vi "update two devices.vi"(0 "VISA resource name":refnum<visa-resource-name>, 7 "Firmware file for Master":path, 11 "Firmware file for Screen":path) -> (15 "error out":errorcluster)   [LabVIEW 2010]
uses:
  <vilib>/Instr/_visa.llb/VISA Configure Serial Port (Instr).vi
panel:
  out "Slide 2":dbl(slide) scale=0.0..1.0
  out "Pages to program 2":T1(array[cluster])
  out "Slide":dbl(slide) scale=0.0..1.0
  out "Pages to program":T1(array[cluster])
  # "Master's Firmware"
  # "Screen's Firmware"
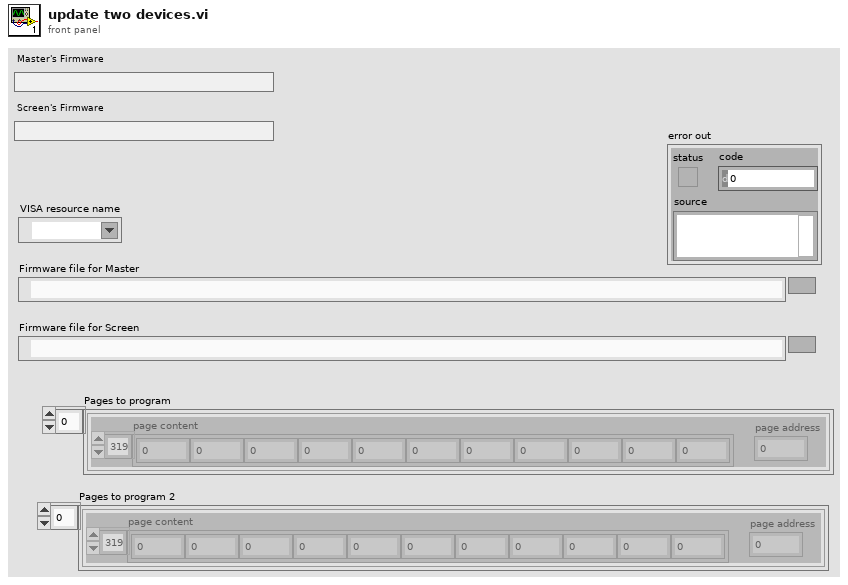
[diagram p1: front panel]
types:
  T1 = cluster{"page content":u8[], "page address":u32}[]
  T2 = cluster{"Byte count":u8, "Address":u16, "Record Type":u8, "Data":u8[], "Checksum":u8, "Start code":string, "Checksum (my)":u8}[]
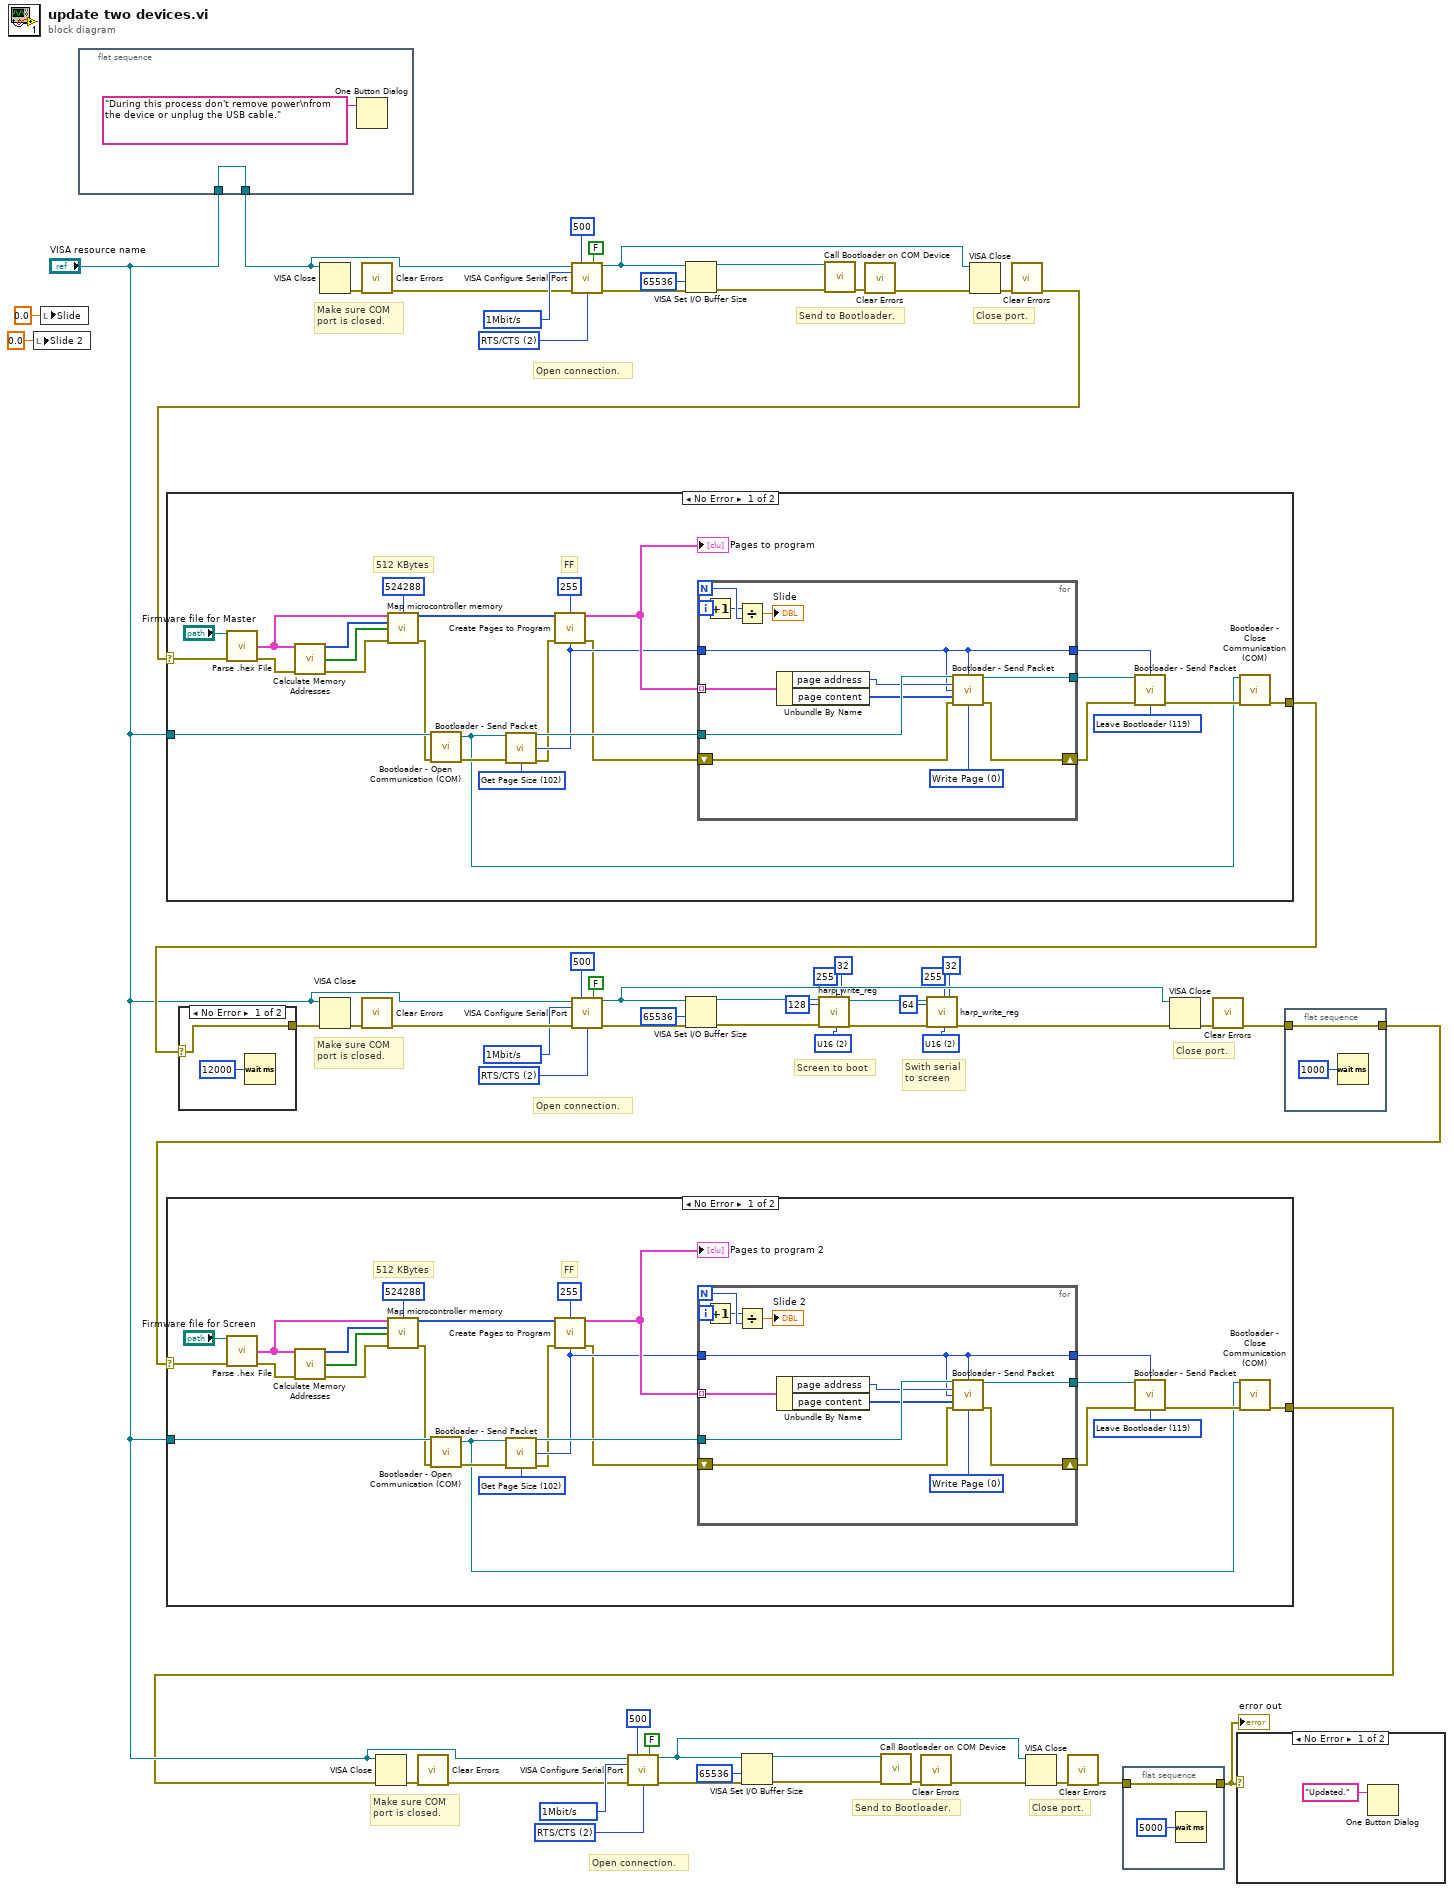
[diagram p0: block diagram]
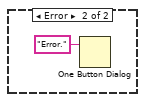
[diagram p3: hidden frame]
diagram:
  w18 = u32 1000000 items=["250Kbit/s"=250000, "500kbit/s"=500000, "1Mbit/s"=1000000, "2Mbit/s"=2000000, "4Mbit/s"=4000000] ("baud rate")
  w19 = u16 2 items=["None", "XON/XOFF", "RTS/CTS", "XON/XOFF & RTS/CTS", "DTR/DSR", "XON/XOFF & DTR/DSR"] ("flow control (0:none)")
  w29 = u8 2 items=["U8"=1, "U16"=2, "U32"=4, "U64"=8, "I8"=129, "I16"=130, "I32"=132, "I64"=136, "FLOAT"=68, "BOOL"=17] ("type")
  w36 = u8 2 items=["U8"=1, "U16"=2, "U32"=4, "U64"=8, "I8"=129, "I16"=130, "I32"=132, "I64"=136, "FLOAT"=68, "BOOL"=17] ("type")
  w43 = u32 1000000 items=["250Kbit/s"=250000, "500kbit/s"=500000, "1Mbit/s"=1000000, "2Mbit/s"=2000000, "4Mbit/s"=4000000] ("baud rate")
  w42 = u16 2 items=["None", "XON/XOFF", "RTS/CTS", "XON/XOFF & RTS/CTS", "DTR/DSR", "XON/XOFF & DTR/DSR"] ("flow control (0:none)")
  w59 = u32 1000000 items=["250Kbit/s"=250000, "500kbit/s"=500000, "1Mbit/s"=1000000, "2Mbit/s"=2000000, "4Mbit/s"=4000000] ("baud rate")
  w60 = u16 2 items=["None", "XON/XOFF", "RTS/CTS", "XON/XOFF & RTS/CTS", "DTR/DSR", "XON/XOFF & DTR/DSR"] ("flow control (0:none)")
  # "Close port."
  # "Send to Bootloader."
  # "Open connection."
  # "Make sure COM\nport is closed."
  # "Screen to boot"
  # "Swith serial\nto screen"
  # "Close port."
  # "Open connection."
  # "Make sure COM\nport is closed."
  # "Close port."
  # "Send to Bootloader."
  # "Open connection."
  # "Make sure COM\nport is closed."
  n1 = local write "Slide 2"(0.0 ("Slide 2")) -> ()
  n2 = local write "Slide"(0.0 ("Slide")) -> ()
  n3 = flat-sequence {
    tunnel: [w64] -> w23
    tunnel: "VISA resource name" -> [w64]
    frame #0 {
      n4 = One Button Dialog(message="During this process don't remove power\nfrom the device or unplug the USB cable.") -> ()  [unwired: 1 in, 1 out]
    }
  }
  n5 = case shown="No Error" w33 {
    selector: w33 -> [w78 w105]
    tunnel: "VISA resource name" -> [w77 _]
    tunnel: [w66 w105] -> w5
    frame No Error {
      w71 = u16 102 items=["Write Page"=0, "Read Page"=1, "Write EEPROM"=2, "Read EEPROM"=3, "Get Page Size"=102, "Leave Bootloader"=119] ("Op Code")
      w87 = u16 119 items=["Write Page"=0, "Read Page"=1, "Write EEPROM"=2, "Read EEPROM"=3, "Check"=102, "Leave Bootloader"=119] ("Op Code")
      # "FF"
      # "512 KBytes"
      n6 = call "Parse .hex File.vi"("file path"="Firmware file for Screen", "error in"=w78) -> (".hex lines"=w81:T2, "error out"=w80:errorcluster)  [unwired: 12 in]
      n7 = call "Calculate Memory Addresses.vi"(".hex lines"=w81, "error in"=w80) -> ("Memory Address"=w82:u32[], "It's a Data Record Type"=w83:bool[], "error out"=w84:errorcluster)  [unwired: 11 in]
      n8 = call "Map microcontroller memory.vi"(".hex lines"=w81, "Memory Max. Size"=524288, "Memory Address"=w82, "It's a Data Record Type"=w83, "error in"=w84) -> ("Complete Memory Map (512KBytes)"=w85:i16[], "error out"=w72:errorcluster)  [unwired: 9 in]
      n9 = call "Bootloader - Open Communication (COM).vi"("COM Port"=w77, "error in (no error)"=w72) -> ("COM Port"=w75:refnum<visa-resource-name>, "error out"=w89:errorcluster)  [unwired: 12 in]
      n10 = call "Bootloader - Send Packet.vi"("VISA resource name"=w75, "error in (no error)"=w89, "Op Code"=w71) -> ("VISA resource name"=w88:refnum<visa-resource-name>, "Data Length"=w70:u32, "error out"=w68:errorcluster)  [unwired: 8 in, 2 out]
      n11 = call "Create Pages to Program.vi"("Complete Memory Map (512KBytes)"=w85, "Memory Default Byte"=u8 255, "error in (no error)"=w68, "Page Size"=w70) -> ("Pages"=w79:T1, "error out"=w67:errorcluster)  [unwired: 10 in]
      "Pages to program 2" <- w79
      n12 = for {
        N -> [w95]
        tunnel: w79 -> [w104] mode=indexing
        tunnel: w88 -> [w103]
        shift-right: [w98] -> w91
        shift-left: w67 -> [w102]
        tunnel: [w97] -> w86
        tunnel: w70 -> [w93]
        tunnel: [w93] -> w69
        i -> [w94]
        w101 = u16 0 items=["Write Page"=0, "Read Page"=1, "Write EEPROM"=2, "Read EEPROM"=3, "Check"=102, "Leave Bootloader"=119] ("Op Code")
        n13 = Increment(x=w94) -> (x+1=w92:i32)
        n14 = Divide(x=w92, y=w95) -> (x/y=→"Slide 2":dbl)
        n15 = Unbundle By Name(w104) -> ("page address"=w100:u32, "page content"=w99:u8[])
        n16 = call "Bootloader - Send Packet.vi"("VISA resource name"=w103, "Data Fixed Length"=w93, "Address"=w100, "Data Length"=w93, "Data"=w99, "error in (no error)"=w102, "Op Code"=w101) -> ("VISA resource name"=w97:refnum<visa-resource-name>, "error out"=w98:errorcluster)  [unwired: 4 in, 3 out]
      }
      n17 = call "Bootloader - Send Packet.vi"("VISA resource name"=w86, "Data Fixed Length"=w69, "error in (no error)"=w91, "Op Code"=w87) -> ("error out"=w90:errorcluster)  [unwired: 7 in, 4 out]
      n18 = call "Bootloader - Close Communication (COM).vi"("COM Port"=w75, "error in (no error)"=w90) -> ("error out"=w66:errorcluster)  [unwired: 13 in]
    }
    frame Error {
    }
  }
  n19 = VISA Close(VISA resource name=w23) -> (error out=w63:errorcluster)  [unwired: 1 in]
  n20 = call <vilib>:"Clear Errors.vi"("error in (no error)"=w63) -> ("error out"=w56:errorcluster)  [unwired: 6 in]
  n21 = VISA Close(VISA resource name="VISA resource name", error in (no error)=w5) -> (error out=w22:errorcluster)
  n22 = call <vilib>:"Clear Errors.vi"("error in (no error)"=w22) -> ("error out"=w15:errorcluster)  [unwired: 6 in]
  n23 = call-poly "VISA Configure Serial Port"("VISA resource name"=w23, "timeout (10sec)"=u32 500, "Enable Termination\nChar (T)"=FALSE ("Enable Termination\nChar (T)"), "baud rate (9600)"=w59, "error in (no error)"=w56, "flow control (0:none)"=w60) -> ("VISA resource name out"=w50:refnum<visa-resource-name>, "error out"=w57:errorcluster)  [unwired: 8 in]
  n24 = call-poly "VISA Configure Serial Port"("VISA resource name"="VISA resource name", "timeout (10sec)"=u32 500, "Enable Termination\nChar (T)"=FALSE ("Enable Termination\nChar (T)"), "baud rate (9600)"=w18, "error in (no error)"=w15, "flow control (0:none)"=w19) -> ("VISA resource name out"=w9:refnum<visa-resource-name>, "error out"=w16:errorcluster)  [unwired: 8 in]
  n25 = VISA Set I/O Buffer Size(VISA resource name=w50, size (4096)=u32 65536, error in (no error)=w57) -> (VISA resource name out=w54:refnum<visa-resource-name>, error out=w55:errorcluster)  [unwired: 1 in]
  n26 = VISA Set I/O Buffer Size(VISA resource name=w9, size (4096)=u32 65536, error in (no error)=w16) -> (VISA resource name out=w13:refnum<visa-resource-name>, error out=w14:errorcluster)  [unwired: 1 in]
  n27 = call "Call Bootloader on COM Device.vi"("port"=w54, "error in (no error)"=w55) -> ("error out"=w52:errorcluster)  [unwired: 12 in, 1 out]
  n28 = call <vilib>:"Clear Errors.vi"("error in (no error)"=w52) -> ("error out"=w51:errorcluster)  [unwired: 6 in]
  n29 = call "Call Bootloader on COM Device.vi"("port"=w13, "error in (no error)"=w14) -> ("error out"=w11:errorcluster)  [unwired: 12 in, 1 out]
  n30 = call <vilib>:"Clear Errors.vi"("error in (no error)"=w11) -> ("error out"=w10:errorcluster)  [unwired: 6 in]
  n31 = VISA Close(VISA resource name=w50, error in (no error)=w51) -> (error out=w53:errorcluster)
  n32 = call <vilib>:"Clear Errors.vi"("error in (no error)"=w53) -> ("error out"=w49:errorcluster)  [unwired: 6 in]
  n33 = case shown="No Error" w49 {
    selector: w49 -> [w118 w145]
    tunnel: "VISA resource name" -> [w117 _]
    tunnel: [w106 w145] -> w32
    frame No Error {
      w111 = u16 102 items=["Write Page"=0, "Read Page"=1, "Write EEPROM"=2, "Read EEPROM"=3, "Get Page Size"=102, "Leave Bootloader"=119] ("Op Code")
      w127 = u16 119 items=["Write Page"=0, "Read Page"=1, "Write EEPROM"=2, "Read EEPROM"=3, "Check"=102, "Leave Bootloader"=119] ("Op Code")
      # "FF"
      # "512 KBytes"
      n34 = call "Parse .hex File.vi"("file path"="Firmware file for Master", "error in"=w118) -> (".hex lines"=w121:T2, "error out"=w120:errorcluster)  [unwired: 12 in]
      n35 = call "Calculate Memory Addresses.vi"(".hex lines"=w121, "error in"=w120) -> ("Memory Address"=w122:u32[], "It's a Data Record Type"=w123:bool[], "error out"=w124:errorcluster)  [unwired: 11 in]
      n36 = call "Map microcontroller memory.vi"(".hex lines"=w121, "Memory Max. Size"=524288, "Memory Address"=w122, "It's a Data Record Type"=w123, "error in"=w124) -> ("Complete Memory Map (512KBytes)"=w125:i16[], "error out"=w112:errorcluster)  [unwired: 9 in]
      n37 = call "Bootloader - Open Communication (COM).vi"("COM Port"=w117, "error in (no error)"=w112) -> ("COM Port"=w115:refnum<visa-resource-name>, "error out"=w129:errorcluster)  [unwired: 12 in]
      n38 = call "Bootloader - Send Packet.vi"("VISA resource name"=w115, "error in (no error)"=w129, "Op Code"=w111) -> ("VISA resource name"=w128:refnum<visa-resource-name>, "Data Length"=w110:u32, "error out"=w108:errorcluster)  [unwired: 8 in, 2 out]
      n39 = call "Create Pages to Program.vi"("Complete Memory Map (512KBytes)"=w125, "Memory Default Byte"=u8 255, "error in (no error)"=w108, "Page Size"=w110) -> ("Pages"=w119:T1, "error out"=w107:errorcluster)  [unwired: 10 in]
      "Pages to program" <- w119
      n40 = for {
        N -> [w135]
        tunnel: w119 -> [w144] mode=indexing
        tunnel: w128 -> [w143]
        shift-right: [w138] -> w131
        shift-left: w107 -> [w142]
        tunnel: [w137] -> w126
        tunnel: w110 -> [w133]
        tunnel: [w133] -> w109
        i -> [w134]
        w141 = u16 0 items=["Write Page"=0, "Read Page"=1, "Write EEPROM"=2, "Read EEPROM"=3, "Check"=102, "Leave Bootloader"=119] ("Op Code")
        n41 = Increment(x=w134) -> (x+1=w132:i32)
        n42 = Divide(x=w132, y=w135) -> (x/y=→"Slide":dbl)
        n43 = Unbundle By Name(w144) -> ("page address"=w140:u32, "page content"=w139:u8[])
        n44 = call "Bootloader - Send Packet.vi"("VISA resource name"=w143, "Data Fixed Length"=w133, "Address"=w140, "Data Length"=w133, "Data"=w139, "error in (no error)"=w142, "Op Code"=w141) -> ("VISA resource name"=w137:refnum<visa-resource-name>, "error out"=w138:errorcluster)  [unwired: 4 in, 3 out]
      }
      n45 = call "Bootloader - Send Packet.vi"("VISA resource name"=w126, "Data Fixed Length"=w109, "error in (no error)"=w131, "Op Code"=w127) -> ("error out"=w130:errorcluster)  [unwired: 7 in, 4 out]
      n46 = call "Bootloader - Close Communication (COM).vi"("COM Port"=w115, "error in (no error)"=w130) -> ("error out"=w106:errorcluster)  [unwired: 13 in]
    }
    frame Error {
    }
  }
  n47 = case shown="No Error" w32 {
    selector: w32 -> [w146 w148]
    tunnel: [w146 w148] -> w31
    frame No Error {
      n48 = Wait (ms)(milliseconds to wait=u32 12000) -> ()  [unwired: 1 out]
    }
    frame Error {
    }
  }
  n49 = VISA Close(VISA resource name="VISA resource name", error in (no error)=w31) -> (error out=w39:errorcluster)
  n50 = call <vilib>:"Clear Errors.vi"("error in (no error)"=w39) -> ("error out"=w46:errorcluster)  [unwired: 6 in]
  n51 = call-poly "VISA Configure Serial Port"("VISA resource name"="VISA resource name", "timeout (10sec)"=u32 500, "Enable Termination\nChar (T)"=FALSE ("Enable Termination\nChar (T)"), "baud rate (9600)"=w43, "error in (no error)"=w46, "flow control (0:none)"=w42) -> ("VISA resource name out"=w48:refnum<visa-resource-name>, "error out"=w45:errorcluster)  [unwired: 8 in]
  n52 = VISA Set I/O Buffer Size(VISA resource name=w48, size (4096)=u32 65536, error in (no error)=w45) -> (VISA resource name out=w38:refnum<visa-resource-name>, error out=w1:errorcluster)  [unwired: 1 in]
  n53 = call "harp_write_reg.vi"(0:"port"=w38, "16 bits"=u16 128, "error in (no error)"=w1, 10:"port"=u8 255 ("port"), "type"=w29, "reg. address"=u8 32) -> ("port out"=w35:refnum<visa-resource-name>, "error out"=w2:errorcluster)  [unwired: 11 in, 1 out]
  n54 = call "harp_write_reg.vi"(0:"port"=w35, "16 bits"=u16 64, "error in (no error)"=w2, 10:"port"=u8 255 ("port"), "type"=w36, "reg. address"=u8 32) -> ("error out"=w30:errorcluster)  [unwired: 11 in, 2 out]
  n55 = VISA Close(VISA resource name=w9, error in (no error)=w10) -> (error out=w12:errorcluster)
  n56 = call <vilib>:"Clear Errors.vi"("error in (no error)"=w12) -> ("error out"=w7:errorcluster)  [unwired: 6 in]
  n57 = flat-sequence {
    tunnel: w7 -> [w149]
    tunnel: [w149] -> w6
    frame #0 {
      n58 = Wait (ms)(milliseconds to wait=u32 5000) -> ()  [unwired: 1 out]
    }
  }
  n59 = VISA Close(VISA resource name=w48, error in (no error)=w30) -> (error out=w47:errorcluster)
  n60 = call <vilib>:"Clear Errors.vi"("error in (no error)"=w47) -> ("error out"=w34:errorcluster)  [unwired: 6 in]
  n61 = case shown="No Error" w6 {
    frame No Error {
      n62 = One Button Dialog(message="Updated.") -> ()  [unwired: 1 in, 1 out]
    }
    frame Error {
      n63 = One Button Dialog(message="Error.") -> ()  [unwired: 1 in, 1 out]
    }
  }
  n64 = flat-sequence {
    tunnel: w34 -> [w153]
    tunnel: [w153] -> w33
    frame #0 {
      n65 = Wait (ms)(milliseconds to wait=u32 1000) -> ()  [unwired: 1 out]
    }
  }
  "error out" <- w6
